vi "ALLPROPS0dll.vi"(8 "error in (no error)":errorcluster, 11 "Inputs":T2) -> (0 "error out":errorcluster, 3 "Outputs":T1)   [LabVIEW 2016]
uses:
  REFPROP.DLL
panel:
  # "REFPROP-ALLPROPS0dll.vi"
  # "void ALLPROPS0dll(int *iIn, int *iOut/* 200 */, int *iFlag, double *T, double *D, double *z/* 20 */, double *Output/* 200 */, int *ierr, char *herr, int herr_length/* 255 */);"
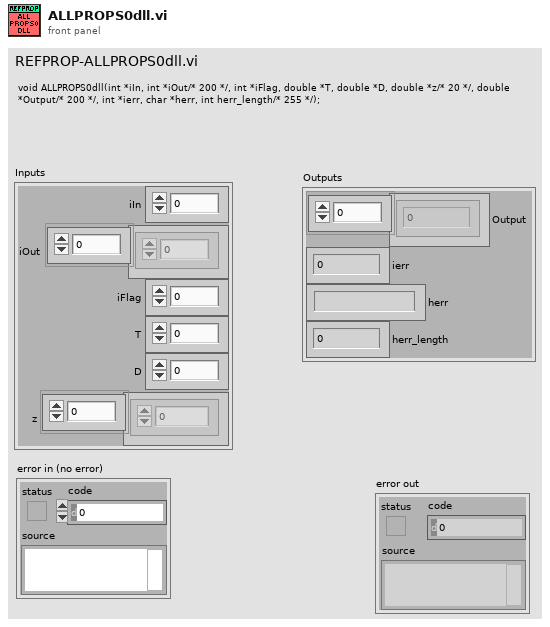
[diagram p1: front panel]
types:
  T1 = cluster{"Output":dbl[], "ierr":i32, "herr":string, "herr_length":i32}
  T2 = cluster{"iIn":i32, "iOut":i32[], "iFlag":i32, "T":dbl, "D":dbl, "z":dbl[]}
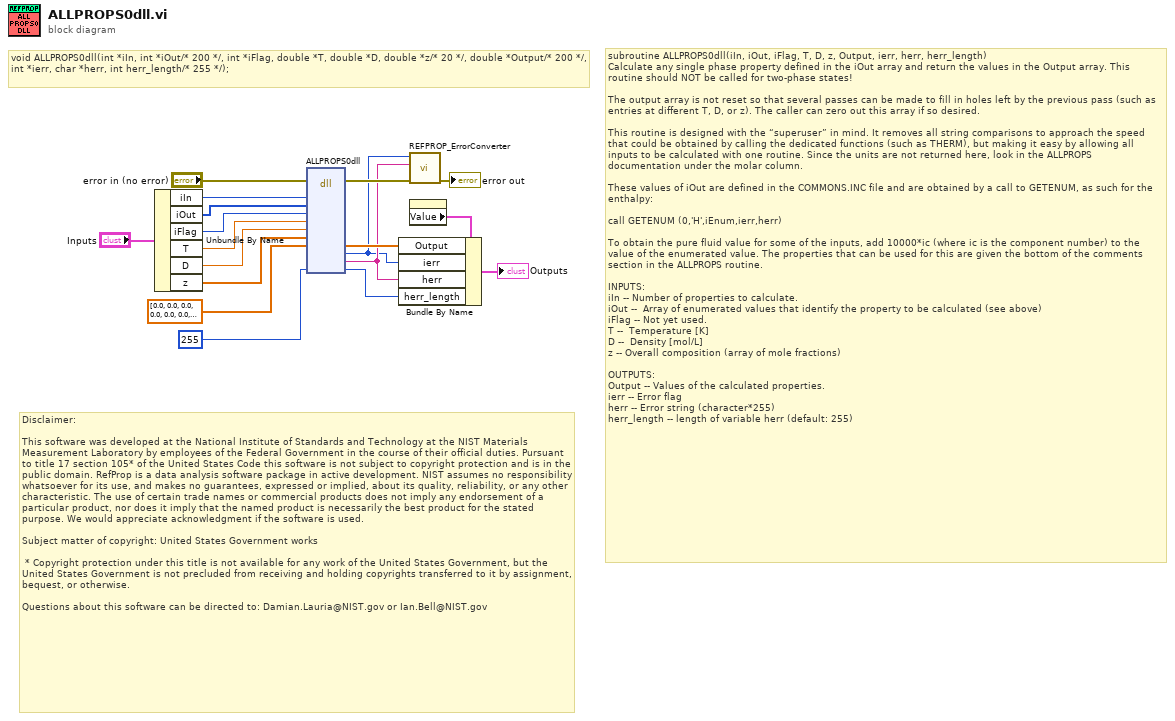
[diagram p0: block diagram]
diagram:
  # "void ALLPROPS0dll(int *iIn, int *iOut/* 200 */, int *iFlag, double *T, double *D, double *z/* 20 */, double *Output/* 200 */, int *ierr, char *herr, int herr_length/* 255 */);"
  # "Disclaimer:\n\nThis software was developed at the National Institute of Standards and Technology at the NIST Materials Measurement Laboratory by employees of the Federal Government in the course of their official duties. Pursuant to title 17 section 105* of the United States Code this software is not subject to copyright protection and is in the public domain. RefProp is a data analysis software package in active development. NIST assumes no responsibility whatsoever for its use, and makes no guarantees, expressed or implied, about its quality, reliability, or any other characteristic. The use of certain trade names or commercial products does not imply any endorsement of a particular product, nor does it imply that the named product is necessarily the best product for the stated purpose. We would appreciate acknowledgment if the software is used.\n \nSubject matter of copyright: United States Government works\n  \n * Copyright protection under this title is not available for any work of the United States Government, but the United States Government is not precluded from receiving and holding copyrights transferred to it by assignment, bequest, or otherwise.\n\nQuestions about this software can be directed to: Damian.Lauria@NIST.gov or Ian.Bell@NIST.gov"
  # "subroutine ALLPROPS0dll(iIn, iOut, iFlag, T, D, z, Output, ierr, herr, herr_length)\nCalculate any single phase property defined in the iOut array and return the values in the Output array. This routine should NOT be called for two-phase states!\n\nThe output array is not reset so that several passes can be made to fill in holes left by the previous pass (such as entries at different T, D, or z). The caller can zero out this array if so desired.\n\nThis routine is designed with the “superuser” in mind. It removes all string comparisons to approach the speed that could be obtained by calling the dedicated functions (such as THERM), but making it easy by allowing all inputs to be calculated with one routine. Since the units are not returned here, look in the ALLPROPS documentation under the molar column.\n\nThese values of iOut are defined in the COMMONS.INC file and are obtained by a call to GETENUM, as such for the enthalpy:\n\ncall GETENUM (0,'H',iEnum,ierr,herr)\n\nTo obtain the pure fluid value for some of the inputs, add 10000*ic (where ic is the component number) to the value of the enumerated value. The properties that can be used for this are given the bottom of the comments section in the ALLPROPS routine.\n\nINPUTS:\t\niIn -- Number of properties to calculate.\niOut --  Array of enumerated values that identify the property to be calculated (see above)\niFlag -- Not yet used.\nT --  Temperature [K]\nD --  Density [mol/L]\nz -- Overall composition (array of mole fractions)\n\nOUTPUTS:\nOutput -- Values of the calculated properties.\nierr -- Error flag\nherr -- Error string (character*255)\nherr_length -- length of variable herr (default: 255)"
  n1 = Unbundle By Name("Inputs") -> ("iIn"=w16:i32, "iOut"=w15:i32[], "iFlag"=w14:i32, "T"=w13:dbl, "D"=w12:dbl, "z"=w11:dbl[])
  n2 = dll-call lib="S:/009 - Testing/02 - Performance Testing/REFPROP/REFPROP.*" fn="ALLPROPS0dll"(error in="error in (no error)", "iIn"=w16, "iOut"=w15, "iFlag"=w14, "T"=w13, "D"=w12, "z"=w11, "Output"=dbl[] [0.0, 0.0, 0.0, 0.0, 0.0, 0.0, 0.0, 0.0, 0.0, 0.0, 0.0, 0.0, 0.0, 0.0, 0.0, 0.0, 0.0, 0.0, 0.0, 0.0, 0.0, 0.0, 0.0, 0.0, 0.0, 0.0, 0.0, 0.0, 0.0, 0.0, 0.0, 0.0, 0.0, 0.0, 0.0, 0.0, 0.0, 0.0, 0.0, 0.0, 0.0, 0.0, 0.0, 0.0, 0.0, 0.0, 0.0, 0.0, 0.0, 0.0, 0.0, 0.0, 0.0, 0.0, 0.0, 0.0, 0.0, 0.0, 0.0, 0.0, 0.0, 0.0, 0.0, 0.0, 0.0, 0.0, 0.0, 0.0, 0.0, 0.0, 0.0, 0.0, 0.0, 0.0, 0.0, 0.0, 0.0, 0.0, 0.0, 0.0, 0.0, 0.0, 0.0, 0.0, 0.0, 0.0, 0.0, 0.0, 0.0, 0.0, 0.0, 0.0, 0.0, 0.0, 0.0, 0.0, 0.0, 0.0, 0.0, 0.0, 0.0, 0.0, 0.0, 0.0, 0.0, 0.0, 0.0, 0.0, 0.0, 0.0, 0.0, 0.0, 0.0, 0.0, 0.0, 0.0, 0.0, 0.0, 0.0, 0.0, 0.0, 0.0, 0.0, 0.0, 0.0, 0.0, 0.0, 0.0, 0.0, 0.0, 0.0, 0.0, 0.0, 0.0, 0.0, 0.0, 0.0, 0.0, 0.0, 0.0, 0.0, 0.0, 0.0, 0.0, 0.0, 0.0, 0.0, 0.0, 0.0, 0.0, 0.0, 0.0, 0.0, 0.0, 0.0, 0.0, 0.0, 0.0, 0.0, 0.0, 0.0, 0.0, 0.0, 0.0, 0.0, 0.0, 0.0, 0.0, 0.0, 0.0, 0.0, 0.0, 0.0, 0.0, 0.0, 0.0, 0.0, 0.0, 0.0, 0.0, 0.0, 0.0, 0.0, 0.0, 0.0, 0.0, 0.0, 0.0, 0.0, 0.0, 0.0, 0.0, 0.0, 0.0, 0.0, 0.0, 0.0, 0.0, 0.0, 0.0], "herr_length"=255) -> (error out=w8:errorcluster, "Output"=w3:dbl[], "ierr"=w1:i32, "herr"=w2:string, "herr_length"=w4:u32)  [unwired: 11 in, 1 out]
  n3 = call "REFPROP_ErrorConverter.vi"("error in (no error)"=w8, "Error Message"=w2, "Error Code"=w1) -> ("error out"=→"error out":errorcluster)  [unwired: 8 in]
  n4 = property on="Outputs" class="Clust (strict)"() -> ("Value"=w5:T1)  [unwired: 2 in, 2 out]
  n5 = Bundle By Name(cluster=w5, "Output"=w3, "ierr"=w1, "herr"=w2, "herr_length"=w4) -> (→"Outputs":T1)
